vi "check_conn2.vi"(1 "error IO":errorcluster) -> (0 "error out":errorcluster)   [LabVIEW 2010]
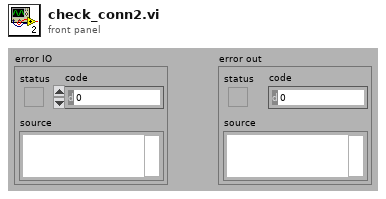
[diagram p1: front panel]
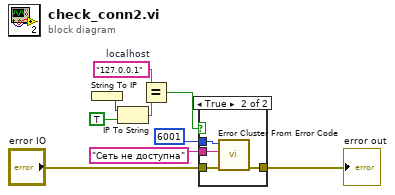
[diagram p0: block diagram]
diagram:
  w2 = "127.0.0.1"  # localhost
  n1 = String To IP() -> (0:w4:u32)  [unwired: 1 in]
  n2 = IP To String(1:TRUE ("dot notation? (F)"), 2:w4) -> (0:w1:string)
  n3 = Equal?(x=w2, y=w1) -> (x = y?=w7:bool)
  n4 = case shown="True" w7 {
    tunnel: "Сеть не доступна" ("string") -> [_ w14]
    tunnel: 6001 ("error code (0)") -> [_ w13]
    tunnel: "error IO" -> [w10 w12]
    tunnel: [w10 w11] -> w9
    frame False {
    }
    frame True {
      n5 = call <vilib>:"Error Cluster From Error Code.vi"("error in (no error)"=w12, "error message (\"\")"=w14, "error code (0)"=w13) -> ("error out"=w11:errorcluster)  [unwired: 6 in]
    }
  }
  "error out" <- w9
